vi "Remove First Slash.vi"(11 "Section":string) -> (3 "result string":string)   [LabVIEW 2022 SP3, in "hse-config.lvlib" / "config-base.lvclass"]
doc: "The \"String to Array\" can't handle a seperation character (slash) as first element. This function removes a leading slash (\"/\") in \"String In\".\n\n____\nHAMPEL SOFTWARE ENGINEERING v3.8.0 (2023-12-18 14:41)"
uses:
  config-base.lvclass
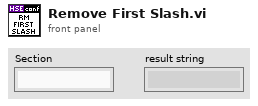
[diagram p1: front panel]
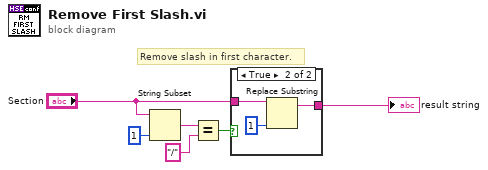
[diagram p0: block diagram]
diagram:
  # "Remove slash in first character."
  n1 = String Subset(string="Section", length (rest)=1 ("length (rest)")) -> (substring=w2:string)  [unwired: 1 in]
  n2 = Equal?(x=w2, y="/") -> (x = y?=w4:bool)
  n3 = case shown="True" w4 {
    tunnel: "Section" -> [w7 w10]
    tunnel: [w7 w8] -> w5
    frame False {
    }
    frame True {
      n4 = Replace Substring(2:1 ("length (len. of substring)"), 5:w10) -> (1:w8:string)  [unwired: 2 in, 1 out]
    }
  }
  "result string" <- w5
